vi "receiveWaveform.vi"(0 "connection ID":refnum<k5>, 1 "error in":errorcluster) -> (2 "signal":waveform(dbl), 3 "connection ID out":refnum<k5>, 4 "error out":errorcluster)   [LabVIEW 2023]
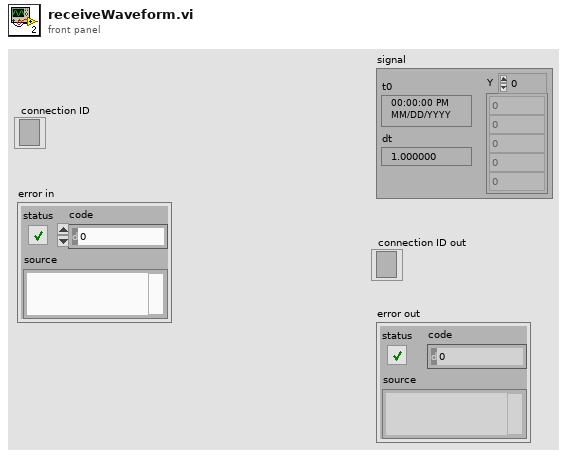
[diagram p1: front panel]
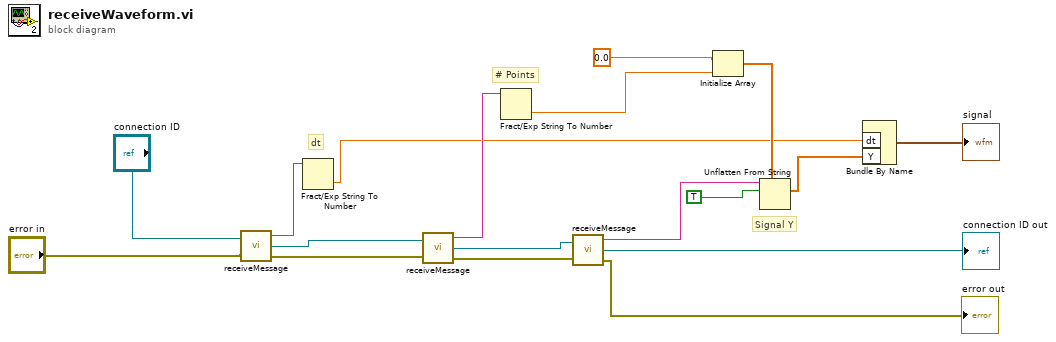
[diagram p0: block diagram]
diagram:
  # "Signal Y"
  # "# Points"
  # "dt"
  n1 = call "receiveMessage.vi"("connection ID"="connection ID", "error in"="error in") -> ("data out"=w16:string, "connection ID out"=w15:refnum<k5>, "error out"=w14:errorcluster)
  n2 = Fract/Exp String To Number(string=w16) -> (number=w5:dbl)  [unwired: 3 in, 1 out]
  n3 = call "receiveMessage.vi"("connection ID"=w15, "error in"=w14) -> ("data out"=w11:string, "connection ID out"=w12:refnum<k5>, "error out"=w13:errorcluster)
  n4 = Fract/Exp String To Number(string=w11) -> (number=w9:dbl)  [unwired: 3 in, 1 out]
  n5 = call "receiveMessage.vi"("connection ID"=w12, "error in"=w13) -> ("data out"=w10:string, "connection ID out"=→"connection ID out":refnum<k5>, "error out"=→"error out":errorcluster)
  n6 = Initialize Array(0.0 ("element"), w9) -> (w7:dbl[])
  n7 = Unflatten From String(type=w7, binary string=w10, data includes array or string size? (T)=TRUE) -> (value=w4:dbl[])  [unwired: 2 in, 2 out]
  n8 = Bundle By Name("dt"=w5, "Y"=w4) -> (→"signal":waveform(dbl))  [unwired: 1 in]
